vi "1D String.vi"(4 "column vector (F)":bool, 7 "key description":string, 8 "sections":string[](array[string]), 9 "string":string[](array[string]), 11 "info data":string) -> (0 "sections out":string[](array[string]), 3 "info data out":string)   [LabVIEW 2013, in "infolib.lvlib"]
doc: "Add a new string table to Info Data string. If section exists in Info Data string, inserts key into this section."
uses:
  infolib.lvlib
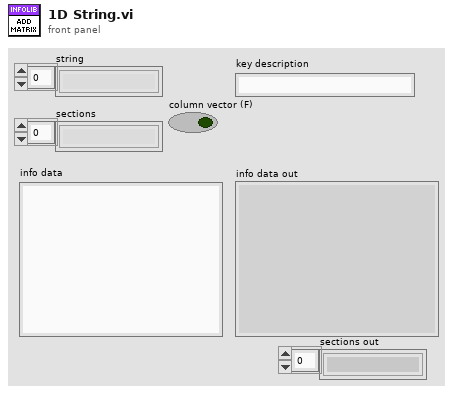
[diagram p1: front panel]
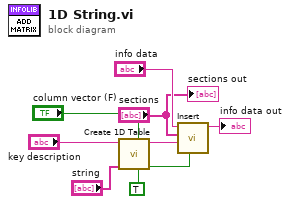
[diagram p0: block diagram]
diagram:
  n1 = call "Create 1D Table.vi"("use apostrophes (F)"=TRUE ("use apostrophes"), "column vector (F)"="column vector (F)", "formatted values"="string", "table name"="key description") -> ("can be indented?"=w2:bool, "table"=w5:string)  [unwired: 6 in]
  n2 = call "Insert.vi"("can be indented? (T)"=w2, "insert"=w5, "sections"="sections", "info data"="info data") -> ("info data out"=→"info data out":string)  [unwired: 7 in]
  "sections out" <- "sections"
